vi "SetHasckelAO.vi"(0 "FPGA API in":refnum<class "FPGA API Concrete.lvclass">, 5 "Haskel in":dbl, 11 "error in (no error)":errorcluster) -> (4 "FPGA API out":refnum<class "FPGA API Concrete.lvclass">, 15 "error out":errorcluster)   [LabVIEW 2019, in "FPGA API Concrete.lvclass"]
uses:
  FPGA API Concrete.lvclass
  FPGA API Concrete.lvclass/FPGA API Concrete.ctl
  <vilib>/Utility/error.llb/Error Cluster From Error Code.vi
  <vilib>/rvi/errors/niLvFpgaAdjustHostInterfaceError.vi
  <vilib>/rvi/interface/nirviReadWriteControl/nirviReadWriteControl.xnode
  FPGA Ref.ctl
  NiFpgaLv.dll
  <vilib>/rvi/interface/Simulation/niFpgaSimulationCallBeginRW.vi
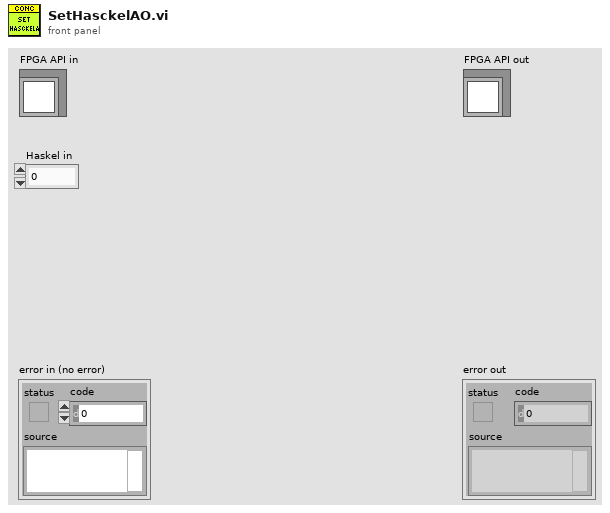
[diagram p1: front panel]
types:
  T1 = typedef "FPGA API Concrete.lvclass/FPGA Ref.ctl" = refnum<k20>
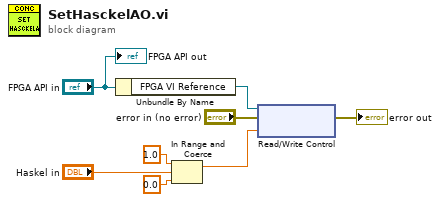
[diagram p0: block diagram]
diagram:
  n1 = Unbundle By Name("FPGA API in") -> ("FPGA VI Reference"=w7:T1)
  n2 = In Range and Coerce(upper limit=1.0, x="Haskel in", lower limit=0.0) -> (coerced(x)=w4:dbl)  [unwired: 1 out]
  n3 = xnode "Read/Write Control"("FPGA VI Reference In"=w7, "error in"="error in (no error)", "Mod5/AO0"=w4) -> ("error out"=→"error out":errorcluster)  [unwired: 1 out]
  "FPGA API out" <- "FPGA API in"
